vi "Refresh Waveform Channels.vi"(6 "new bitfile dma channels":T1[](array[typedef]) {"Data Type" format="%.0x"}, 8 "error in (no error)":errorcluster, 9 "waveform type GUID":string, 10 "waveform inputs name":string, 11 "item ref in":T3 format="%.0x") -> (0 "error out":errorcluster, 3 "item ref out":T3 format="%.0x")   [LabVIEW 2018, in "FPGA Addon System Explorer.lvlib"]
uses:
  FPGA Addon System Explorer.lvlib
  <vilib>/NI Veristand/Custom Device API/Custom Device Item Ref.ctl
  Addon Shared/Types/DMA Information.ctl
  Addon Shared/Types/Data Type.ctl
  Addon Shared/Types/FG Action.ctl
  <vilib>/NI Veristand/Custom Device Tools/Custom Device Utility Library/NI VeriStand - Search for Item by GUID.vi
  Addon Shared/SubVIs/Constants.vi
  <vilib>/NI/NI VeriStand Advanced SysDef API/SysDef API/SysDef.Property.Get.vi
  <vilib>/NI/NI VeriStand Advanced SysDef API/_SubVIs/SysDef.Property.Get.Variant.vi
  <vilib>/NI/NI VeriStand Advanced SysDef API/SysDef API/SysDef.Property.Set.vi
  <vilib>/NI/NI VeriStand Advanced SysDef API/_SubVIs/SysDef.Property.Set.Variant.vi
  Addon Shared/FPGA Addon Shared.lvlib
  <vilib>/NI Veristand/Custom Device Tools/Custom Device Utility Library/Custom Device Utility Library.lvlib
  <vilib>/NI Veristand/Custom Device API/Custom Device API.lvlib
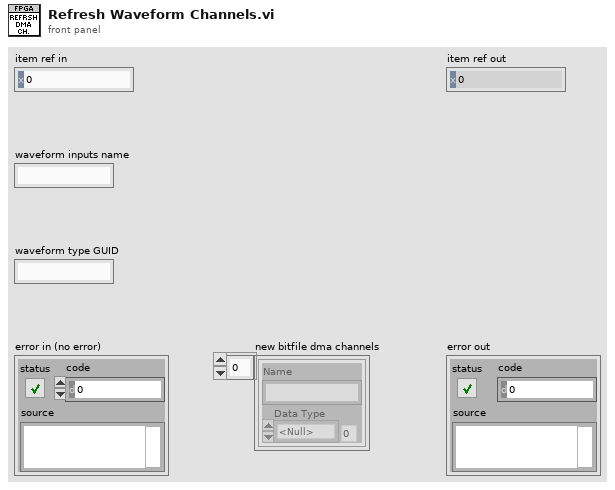
[diagram p1: front panel]
types:
  T1 = typedef "FPGA Addon Shared.lvlib/DMA Information.ctl" = cluster{"Name":string, "Data Type":T2}
  T2 = typedef "FPGA Addon Shared.lvlib/Data Type.ctl" = enum8{"<Null>", "I8", "I16", "I32", "I64", "U8", "U16", "U32", "U64", "SGL", "Boolean", "Analog PWM In Settings", "Analog PWM In", "Digital PWM In Settings", "Digital PWM In", "Digital PWM Out", "Sine Out", "FXP+/-24.5", "FXP+/-16.5", "FXP+/-32.8", "FXP+/-64.32", "FXP+/-16.7", "FXP+/-20.5", "FXP+/-27.5", "FXP+/-32.16", "FXP+16.3", "FXP+18.3", "Digital Static In", "Digital Static Out", "Digital Static In Settings", "Digital WSS Out", "Quad Encoder Settings", "Quad Encoder In", "Group"}
  T3 = typedef "Custom Device API.lvlib/Custom Device Item Ref.ctl" = u64
  T4 = typedef "FPGA Addon Shared.lvlib/FG Action.ctl" = enum8{"GET", "SET"}
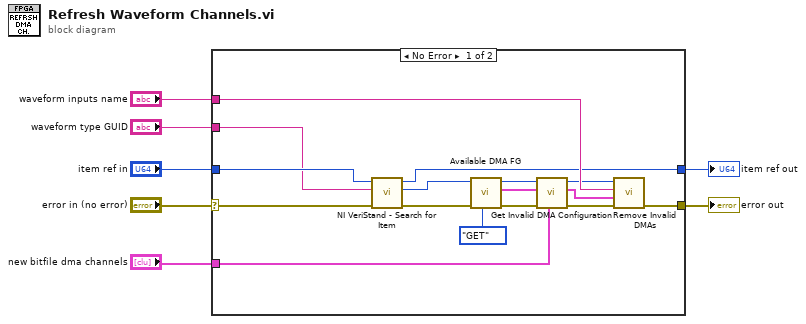
[diagram p0: block diagram]
diagram:
  n1 = case shown="No Error" "error in (no error)" {
    selector: "error in (no error)" -> [w8 w25]
    tunnel: "item ref in" -> [w23 w24]
    tunnel: [w22 w25] -> w6
    tunnel: "waveform type GUID" -> [w16 _]
    tunnel: "waveform inputs name" -> [w15 _]
    tunnel: "new bitfile dma channels" -> [w12 _]
    tunnel: [w10 w24] -> w2
    frame No Error {
      n2 = call-poly <vilib>:"NI VeriStand - Search for Item.vi"("error in"=w8, "Item GUID"=w16, "Section Ref in"=w23) -> ("error out"=w18:errorcluster, "Item Ref"=w17:T3, "Section Ref out"=w10:T3)  [unwired: 5 in, 1 out]
      n3 = call "Available DMA FG.vi"("Action"=FG_Action."GET", "error in (no error)"=w18, "Item Ref"=w17) -> ("error out"=w19:errorcluster, "Available DMA"=w13:T1[], "Item Ref out"=w14:T3)  [unwired: 6 in]
      n4 = call "Get Invalid DMA Configuration.vi"("new bitfile dma channels"=w12, "error in (no error)"=w19, "old bitfile dma channels"=w13, "item ref in"=w14) -> ("error out"=w21:errorcluster, "invalid dma data channels"=w9:T1[], "item ref out"=w11:T3)  [unwired: 5 in]
      n5 = call "Remove Invalid DMAs.vi"("error in (no error)"=w21, "invalid DMA channels"=w9, "section name"=w15, "item ref in"=w11) -> ("error out"=w22:errorcluster)  [unwired: 6 in, 1 out]
    }
    frame Error {
    }
  }
  "item ref out" <- w2
  "error out" <- w6
